vi "CalcDistance.vi"(11 "Reset Encoders":bool) -> (1 "CM Vasen":dbl, 2 "CM Taka":dbl, 3 "CM Etu":dbl, 4 "CM Oikea":dbl)   [LabVIEW 2018]
uses:
  <vilib>/myRIO/Common/Instrument Driver Framework/myRIO v1.0/Encoder/typedefs/Encoder Signal Mode.ctl
  <vilib>/myRIO/Instrument Drivers/Onboard IO/Encoder/typedefs/Encoder Reference.ctl
  <vilib>/myRIO/Common/Instrument Driver Framework/Utilities/typedefs/myRIO Generic Hardware Reference.ctl
  <vilib>/myRIO/Common/Instrument Driver Framework/Utilities/typedefs/Hardware Version Enum.ctl
  <vilib>/myRIO/Common/Instrument Driver Framework/Utilities/typedefs/myRIO v1.0 Reference.ctl
  <vilib>/myRIO/Common/Instrument Driver Framework/Utilities/typedefs/Generic FPGA Reference.ctl
  <vilib>/myRIO/Common/Instrument Driver Framework/myRIO v1.0/Encoder/typedefs/Encoder Channels Enum.ctl
  <vilib>/myRIO/Common/Instrument Driver Framework/myRIO v1.0/Encoder/typedefs/Encoder Configuration v1.0.ctl
  <vilib>/userdefined/High Color/nirio_resource_hc.ctl
  <vilib>/myRIO/Common/Instrument Driver Framework/Utilities/vis/Is FPGA Ref Available.vi
  <vilib>/myRIO/Common/Instrument Driver Framework/myRIO v1.0/Encoder/vis/myRIO v1.1 Open Encoder.vi
  <vilib>/myRIO/Instrument Drivers/Onboard IO/Encoder/vis/Read.vi
  <vilib>/myRIO/Common/Instrument Driver Framework/Utilities/vis/Validate Channels.vi
  <vilib>/myRIO/Common/Instrument Driver Framework/myRIO v1.0/Encoder/vis/myRIO v1.0 Reserve Encoder.vi
  <vilib>/myRIO/Common/Instrument Driver Framework/myRIO v1.0/Encoder/vis/myRIO v1.0 Build MUX Configuration Encoder.vi
  <vilib>/myRIO/Common/Instrument Driver Framework/myRIO v1.0/Resource Manager/vis/myRIO v1.0 Reserve Channel List.vi
  <vilib>/myRIO/Common/Instrument Driver Framework/myRIO v1.0/Resource Manager/vis/myRIO v1.0 Create Configuration List.vi
  <vilib>/myRIO/Common/Instrument Driver Framework/myRIO v1.0/Resource Manager/vis/myRIO v1.0 Reserve Channel.vi
  <vilib>/myRIO/Common/Instrument Driver Framework/myRIO v1.0/Resource Manager/vis/myRIO v1.0 Unreserve Channel.vi
  <vilib>/myRIO/Common/Instrument Driver Framework/myRIO v1.0/Resource Manager/vis/myRIO v1.0 Build Mutex Name.vi
  <vilib>/Utility/VariantDataType/GetNumericInfo.vi
  <vilib>/Utility/error.llb/Error Cluster From Error Code.vi
  <vilib>/myRIO/Common/Instrument Driver Framework/myRIO v1.0/myRIO v1.1 Open.vi
  <vilib>/myRIO/Common/Instrument Driver Framework/Utilities/vis/IO Manager.vi
  <vilib>/myRIO/Common/Instrument Driver Framework/Utilities/vis/Configuration Manager.vi
  <vilib>/myRIO/Common/Instrument Driver Framework/myRIO v1.0/Resource Manager/vis/myRIO v1.0 Configure IO.vi
  <vilib>/myRIO/Common/Instrument Driver Framework/myRIO v1.0/myRIO v1.0 Close.vi
  <vilib>/myRIO/Common/Instrument Driver Framework/myRIO v1.0/Encoder/vis/myRIO v1.0 Configure Encoder.vi
  <vilib>/myRIO/Common/Instrument Driver Framework/myRIO v1.0/Encoder/vis/myRIO v1.0 Read Encoder.vi
  <vilib>/myRIO/Express VI/Onboard IO/Encoder/Encoder Express VI.xnode
  <vilib>/myRIO/Instrument Drivers/Onboard IO/Encoder/vis/myRIO Encoder Open.xnode
  <vilib>/myRIO/Common/Instrument Driver Framework/myRIO v1.0/Encoder/typedefs/Encoder Count Direction Enum.ctl
  <vilib>/myRIO/Instrument Drivers/Onboard IO/Encoder/Encoder.lvlib
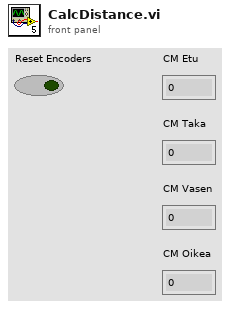
[diagram p1: front panel]
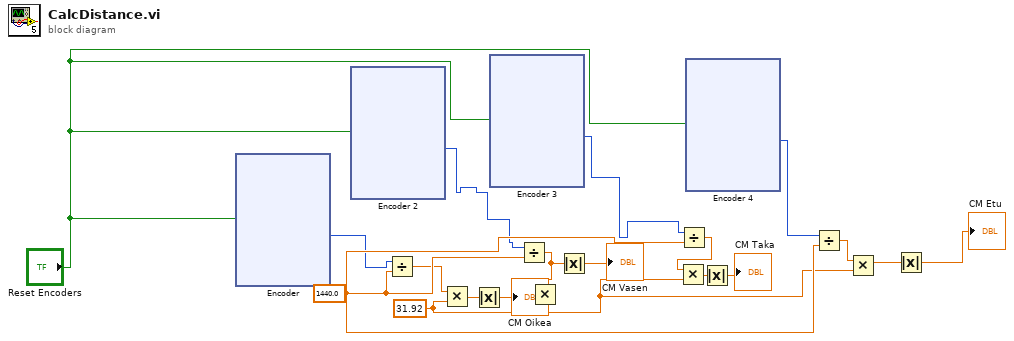
[diagram p0: block diagram]
diagram:
  w18 = 1440.0
  w12 = 31.92
  n1 = xnode "Encoder"("Reset Counter"="Reset Encoders") -> ("Counter Value"=w10:i32)  [unwired: 1 in, 3 out]
  n2 = xnode "Encoder 2"("Reset Counter"="Reset Encoders") -> ("Counter Value"=w15:i32)  [unwired: 1 in, 3 out]
  n3 = Divide(x=w10, y=w18) -> (x/y=w11:dbl)
  n4 = Multiply(x=w11, y=w12) -> (x*y=w1:dbl)
  n5 = Absolute Value(x=w1) -> (abs(x)=→"CM Oikea":dbl)
  n6 = xnode "Encoder 3"("Reset Counter"="Reset Encoders") -> ("Counter Value"=w16:i32)  [unwired: 1 in, 3 out]
  n7 = Divide(x=w15, y=w18) -> (x/y=w3:dbl)
  n8 = Multiply(x=w3, y=w12) -> ()  [unwired: 1 out]
  n9 = Absolute Value(x=w3) -> (abs(x)=→"CM Vasen":dbl)
  n10 = Divide(x=w16, y=w18) -> (x/y=w14:dbl)
  n11 = Multiply(x=w14, y=w12) -> (x*y=w5:dbl)
  n12 = xnode "Encoder 4"("Reset Counter"="Reset Encoders") -> ("Counter Value"=w17:i32)  [unwired: 1 in, 3 out]
  n13 = Absolute Value(x=w5) -> (abs(x)=→"CM Taka":dbl)
  n14 = Divide(x=w17, y=w18) -> (x/y=w13:dbl)
  n15 = Multiply(x=w13, y=w12) -> (x*y=w8:dbl)
  n16 = Absolute Value(x=w8) -> (abs(x)=→"CM Etu":dbl)
